vi "Actor Core.vi"(8 "error in":errorcluster, 11 "Cursor Digitizer in":refnum<class "Cursor Digitizer.lvclass">) -> (0 "error out":errorcluster, 3 "Actor out":refnum<class "Actor.lvclass">)   [LabVIEW 2016, in "Cursor Digitizer.lvclass"]
doc: "(<B>Filename</B>: Actor Framework.lvlib:Actor.lvclass:Actor Core.vi)\n\nReceives messages to the actor, reacts to them, and initiates any error handling that may shut the actor down.\n\nDescendant classes may override this VI to append parallel tasks for the actor to complete while it handles messages. Overrides use the Call Parent Method node."
uses:
  Cursor Digitizer.lvclass
  C:/Program Files/National Instruments/LabVIEW 2016/vi.lib/ActorFramework/Actor/Actor.lvclass
  <vilib>/ActorFramework/Actor/Actor.lvclass
  Cursor Digitizer.lvclass/Cursor Digitizer.ctl
  <vilib>/ActorFramework/Actor/Actor.lvclass/Actor.ctl
  <vilib>/ActorFramework/Message Enqueuer/Message Enqueuer.lvclass/Message Enqueuer.ctl
  Cursor Digitizer Messages/Update Cursor State Msg/Update Cursor State Msg.lvclass/Update Cursor State Msg.ctl
  <vilib>/event_ctls.llb/eventvkey.ctl
  <vilib>/ActorFramework/Message Enqueuer/Init from Existing Queue.vi
  <vilib>/ActorFramework/Message Enqueuer/Enqueue.vi
  Cursor Digitizer Messages/Update Cursor State Msg/Update Cursor State Msg.lvclass
  C:/Program Files/National Instruments/LabVIEW 2016/vi.lib/ActorFramework/Message/Message.lvclass
  Cursor Digitizer Messages/Store XY Msg/Store XY Msg.lvclass
  <vilib>/ActorFramework/Message Priority Queue/Priority Enqueue.vi
  <vilib>/Utility/file.llb/Write Delimited Spreadsheet (DBL).vi
  <vilib>/ActorFramework/Message Enqueuer/Message Enqueuer.lvclass
panel:
  in  "Clear Button":bool
  in  "Save Button":bool
  in  "X-Y values":dbl[][](array[numeric]) format="%#_6p"
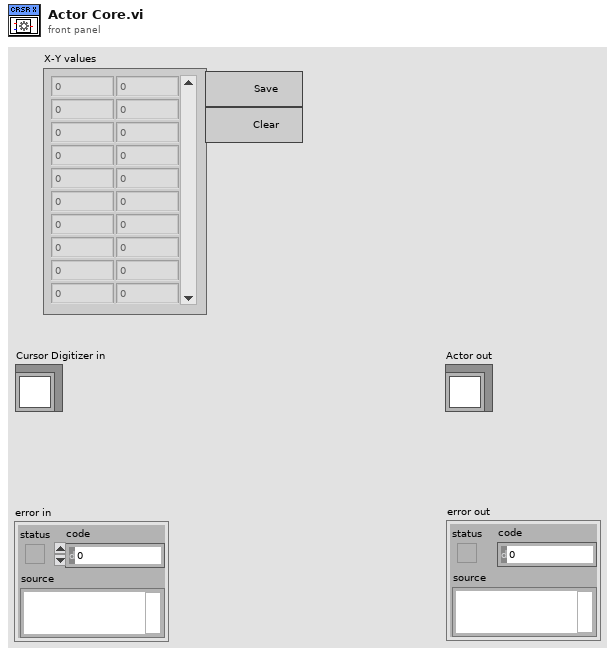
[diagram p1: front panel]
types:
  T1 = typedef "eventvkey.ctl" = enum16{"ASCII", "Enter", "Return", "Shift", "Ctrl", "Alt", "Cmd", "Opt", "Caps", "NumLock", "Clear", "Break", "Up", "Down", "Left", "Right", "Insert", "Delete", "Home", "End", "PageUp", "PageDown", "Escape", "Help", "Pause", "ScrollLock", "F1", "F2", "F3", "F4", "F5", "F6", "F7", "F8", "F9", "F10", "F11", "F12", "F13", "F14", "F15", "F16", "F17", "F18", "F19", "F20", "F21", "F22", "F23", "F24", "Play", "VolumeUp", "VolumeDown", "Mute", "Two Byte Char"}
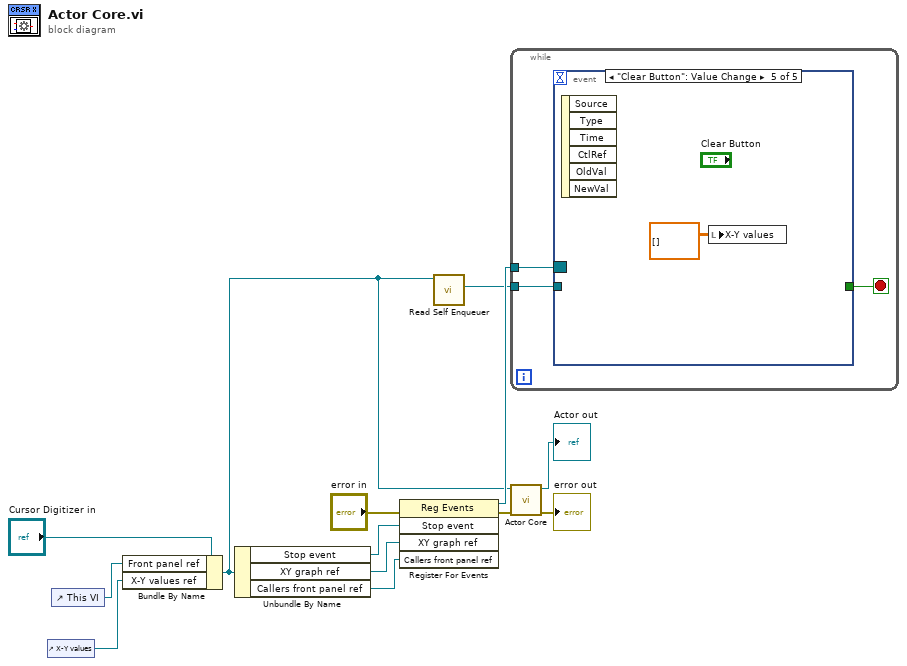
[diagram p0: block diagram]
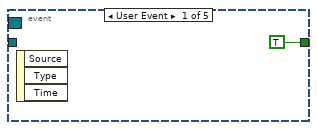
[diagram p2: hidden frame]
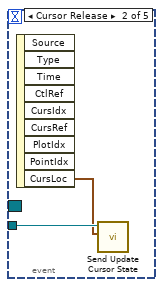
[diagram p3: hidden frame]
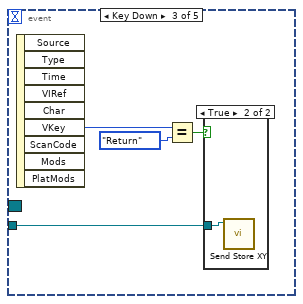
[diagram p4: hidden frame]
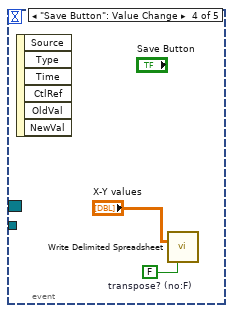
[diagram p6: hidden frame]
diagram:
  n1 = control-ref of="X-Y values"() -> (w1:refnum<vi>)
  n2 = control-ref of="This VI"() -> (w3:refnum<vi>)
  n3 = Bundle By Name(cluster="Cursor Digitizer in", "Front panel ref"=w3, "X-Y values ref"=w1) -> (w5:refnum<class "Cursor Digitizer.lvclass">)
  n4 = Unbundle By Name(w5) -> ("Stop event"=w11:refnum<user-event>, "XY graph ref"=w4:refnum<vi>, "Callers front panel ref"=w2:refnum<vi>)
  n5 = register-events(error in="error in", w11, w4, w2) -> (reference out=w8:refnum<event-registration>, error out=w9:errorcluster)  [unwired: 1 in]
  n6 = call <vilib>:"Read Self Enqueuer.vi"("Actor"=w5) -> ("Self Enqueuer"=w6:refnum<class "Message Enqueuer.lvclass">)  [unwired: 10 in]
  n7 = while {
    tunnel: w8 -> [w16]
    tunnel: w6 -> [w14]
    stop <- w15 stop-if-true
    n8 = event shown="[4] \"Clear Button\": Value Change" {
      selector: w16 -> [_ _ _ _ _]
      dyn-events: _ -> [_ _ _ _ _]
      timeout: _ -> [_ _ _ _ _]
      tunnel: [TRUE _ _ _ _] -> w15
      tunnel: w14 -> [_ w19 w20 _ _]
      event User Event {
        n9 = event-data() -> ()  [unwired: 1 in, 3 out]
      }
      event Cursor Release {
        n10 = event-data() -> ("CursLoc"=w18:cluster{"X":dbl, "Y":dbl})  [unwired: 1 in, 8 out]
        n11 = call "Send Update Cursor State.vi"("Cursor State"=w18, "Message Enqueuer"=w19) -> ()  [unwired: 8 in, 2 out]
      }
      event Key Down {
        n12 = event-data() -> ("VKey"=w23:T1)  [unwired: 1 in, 8 out]
        n13 = Equal?(x=w23, y=eventvkey."Return" ("VKey")) -> (x = y?=w21:bool)
        n14 = case shown="True" w21 {
          tunnel: w20 -> [_ w24]
          frame False {
          }
          frame True {
            n15 = call "Send Store XY.vi"("Message Enqueuer"=w24) -> ()  [unwired: 9 in, 2 out]
          }
        }
      }
      event "Save Button": Value Change {
        w25 = FALSE  # transpose? (no:F)
        n16 = event-data() -> ()  [unwired: 1 in, 6 out]
        n17 = call-poly <vilib>:"Write Delimited Spreadsheet.vi"("2D data"="X-Y values", "transpose? (no:F)"=w25) -> ()  [unwired: 12 in, 2 out]
      }
      event "Clear Button": Value Change {
        n18 = event-data() -> ()  [unwired: 1 in, 6 out]
        n19 = local write "X-Y values"(dbl[][] [] ("X-Y values")) -> ()
      }
    }
  }
  n20 = call-parent "Actor Core.vi"("error in"=w9, "Actor in"=w5) -> ("error out"=→"error out":errorcluster, "Actor out"=→"Actor out":refnum<class "Actor.lvclass">)  [unwired: 8 in]
